vi "Get position API.vi"(8 "Error In":errorcluster) -> (0 "Error Out":errorcluster)   [LabVIEW 2017, in "Colour Wheel.lvlib"]
uses:
  Colour Wheel.lvlib
  Controls/Command Data [cluster].ctl
  Controls/Commands [enum].ctl
  Controls/Params.ctl
  Events/Events.lvlib
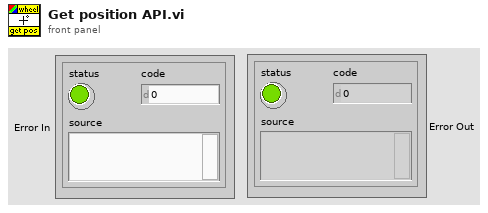
[diagram p1: front panel]
types:
  T1 = typedef "Colour Wheel.lvlib/Params.ctl" = cluster{"Reference":i32, "Colour Wheel Wavelengths":dbl[], "Waveform Index":i32, "COM Port":refnum<visa-resource-name>, "Enabled?":bool}
  T2 = typedef "Colour Wheel.lvlib/Command Data [cluster].ctl" = cluster{"Command":T3, "Data":variant}
  T3 = typedef "Colour Wheel.lvlib/Commands [enum].ctl" = enum16{"Start", "Move", "Get position", "Stop", "Send data"}
  T4 = typedef "Events.lvlib/Refs [cluster].ctl" = cluster{"Exit":refnum<user-event>, "Controller":refnum<user-event>, "System Error":refnum<user-event>, "UI":refnum<user-event>, "Example Module":refnum<user-event>, "Shutter":refnum<user-event>, "Monochromator":refnum<user-event>, "DAQ":refnum<user-event>, "Scope":refnum<user-event>, "Processing":refnum<user-event>, "File IO":refnum<user-event>, "Colour wheel":refnum<user-event>}
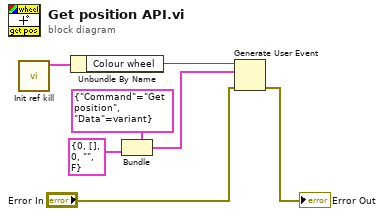
[diagram p0: block diagram]
diagram:
  n1 = call "Init ref kill.vi"() -> ("Messages"=w7:T4)  [unwired: 10 in, 1 out]
  n2 = Unbundle By Name(w7) -> ("Colour wheel"=w6:refnum<user-event>)
  n3 = Bundle(cluster=T2 {"Command"=enum."Get position", "Data"=variant} ("event data"), "Data"=T1 {"Reference"=0, "Colour Wheel Wavelengths"=[], "Waveform Index"=0, "COM Port"="", "Enabled?"=FALSE} ("Monochromator")) -> (w4:T2)  [unwired: 1 in]
  n4 = Generate User Event(user event=w6, event data cluster=w4, error in="Error In") -> (error out=→"Error Out":errorcluster)  [unwired: 1 in, 1 out]
